vi "rs3 run_onchip_tare.vi"(0 "Device in":u64=2008212946240, 1 "Linux/Windows":u16(ring) items=["Linux (poling)", "Windows (interrupt)"], 2 "Auto Depth Preset\n(5 sec slower)":bool, 3 "On-Chip Calibration Mode":u16(ring) items=["Intrinsic", "Extrinsic"], 5 "ground truth, mm":sgl=500.0, 7 "Max step count (5-30)":u16=20, 9 "accuracy":u16(ring) items=["Very High (0.025%)", "High (0.05%)", "Medium (0.1%)", "Low (0.2%)"], 11 "error in (no error)":errorcluster, 12 "average step count (1-30)":u16=10, 13 "timeout ms":i32=8000) -> (4 "Device out":u64=2008212946240, 10 "error":u64, 14 "PointerToNewCalibrationTable":u64=2009804399744, 15 "error out":errorcluster)   [LabVIEW 2017, in "libRealSense3.lvlib"]
doc: "STARTS the streaming of a specific sensor, based on the input QUEUE."
uses:
  libRealSense3.lvlib
  realsense2.dll
panel:
  out "json":string="{\"average step count\": 10,\"step count\": 10, \"accuracy\": 0, \"scan parameter\": 0, \"data sampling\": 0}"
  # "RS Run On-Chip Tare"
  # "(C) 2019 Intel Corp.,  AGJ"
  # "[?1/?16/?2020 8:52 AM]  Angerman, Avishag:  \nstd::stringstream ss;\n        ss << \"{\\n \\\"speed\\\":\" << speed <<\n               \",\\n \\\"average_step_count\\\":\" << average_step_count <<\n               \",\\n \\\"step_count\\\":\" << step_count <<\n               \",\\n \\\"accuracy\\\":\" << accuracy <<\"}\"; \nthis is what I create on viewer , maybe you should try with \\n"
  # "std::stringstream ss;\n        ss << \"{\\n \\\"speed\\\":\" << speed <<\n               \",\\n \\\"average_step_count\\\":\" << average_step_count <<\n               \",\\n \\\"step_count\\\":\" << step_count <<\n               \",\\n \\\"accuracy\\\":\" << accuracy <<\"}\";"
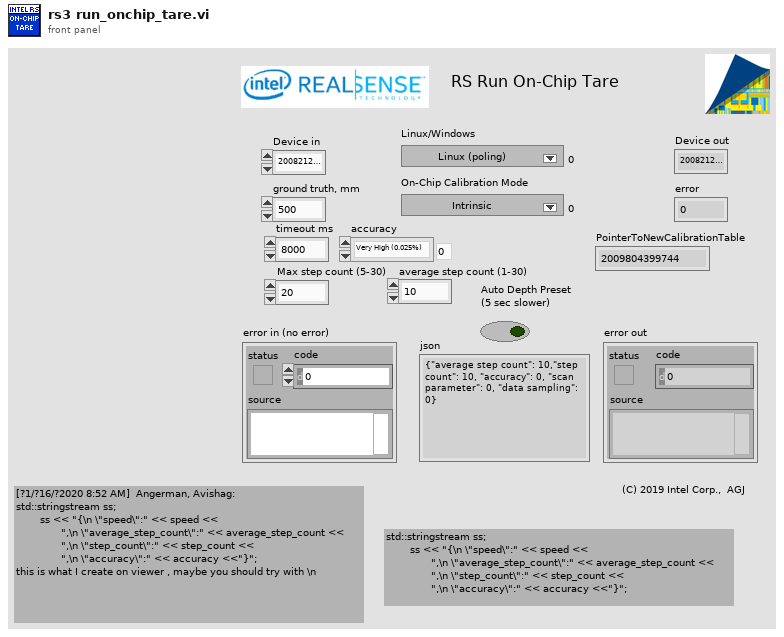
[diagram p1: front panel]
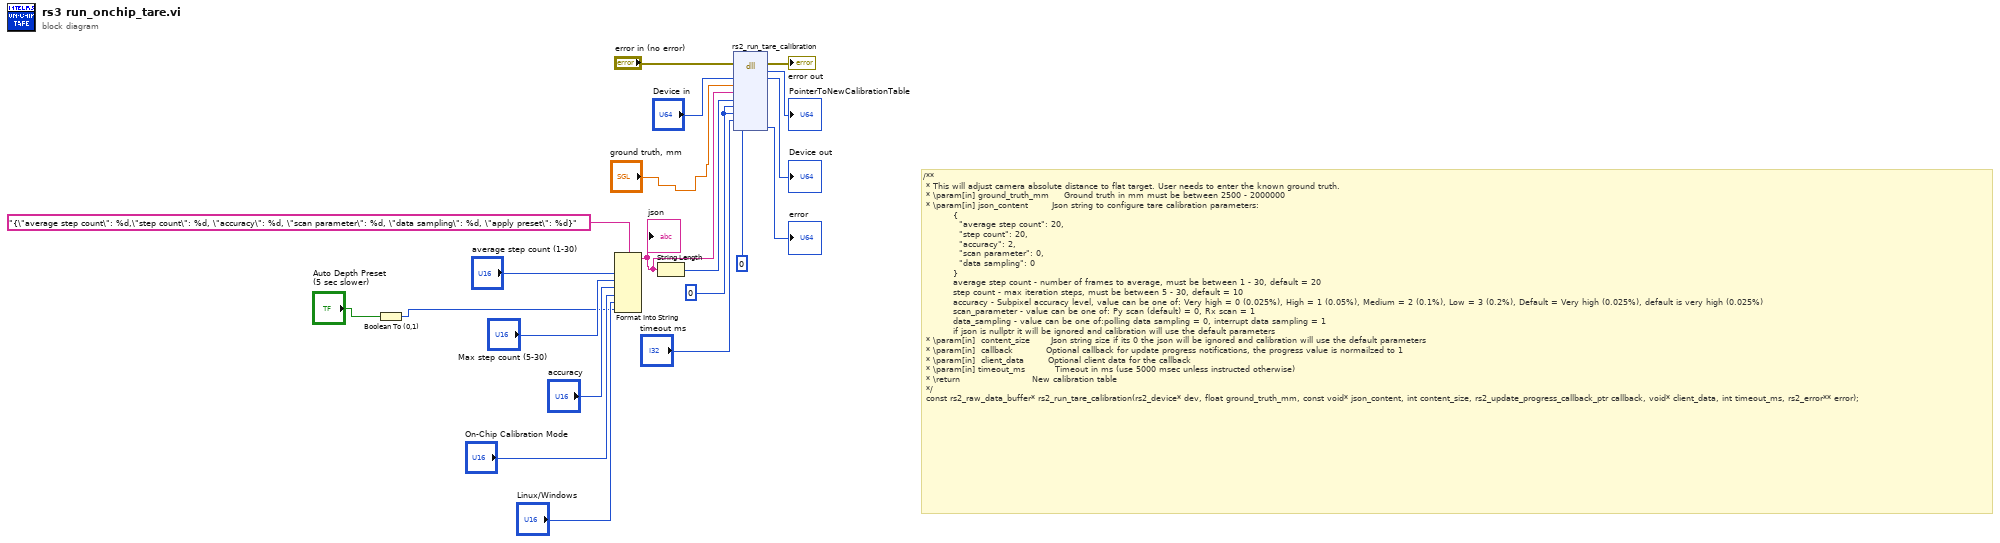
[diagram p0: block diagram]
diagram:
  w10 = u64 0 ("callback progress")
  # "/**\n\t* This will adjust camera absolute distance to flat target. User needs to enter the known ground truth.\n\t* \\param[in] ground_truth_mm     Ground truth in mm must be between 2500 - 2000000\n\t* \\param[in] json_content        Json string to configure tare calibration parameters:\n\t\t\t\t\t\t\t\t\t\t{\n\t\t\t\t\t\t\t\t\t\t  \"average step count\": 20,\n\t\t\t\t\t\t\t\t\t\t  \"step count\": 20,\n\t\t\t\t\t\t\t\t\t\t  \"accuracy\": 2,\n\t\t\t\t\t\t\t\t\t\t  \"scan parameter\": 0,\n\t\t\t\t\t\t\t\t\t\t  \"data sampling\": 0\n\t\t\t\t\t\t\t\t\t\t}\n\t\t\t\t\t\t\t\t\t\taverage step count - number of frames to average, must be between 1 - 30, default = 20\n\t\t\t\t\t\t\t\t\t\tstep count - max iteration steps, must be between 5 - 30, default = 10\n\t\t\t\t\t\t\t\t\t\taccuracy - Subpixel accuracy level, value can be one of: Very high = 0 (0.025%), High = 1 (0.05%), Medium = 2 (0.1%), Low = 3 (0.2%), Default = Very high (0.025%), default is very high (0.025%)\n\t\t\t\t\t\t\t\t\t\tscan_parameter - value can be one of: Py scan (default) = 0, Rx scan = 1\n\t\t\t\t\t\t\t\t\t\tdata_sampling - value can be one of:polling data sampling = 0, interrupt data sampling = 1\n\t\t\t\t\t\t\t\t\t\tif json is nullptr it will be ignored and calibration will use the default parameters\n\t* \\param[in]  content_size       Json string size if its 0 the json will be ignored and calibration will use the default parameters\n\t* \\param[in]  callback           Optional callback for update progress notifications, the progress value is normailzed to 1\n\t* \\param[in]  client_data        Optional client data for the callback\n\t* \\param[in] timeout_ms          Timeout in ms (use 5000 msec unless instructed otherwise)\n\t* \\return                        New calibration table\n\t*/\n\tconst rs2_raw_data_buffer* rs2_run_tare_calibration(rs2_device* dev, float ground_truth_mm, const void* json_content, int content_size, rs2_update_progress_callback_ptr callback, void* client_data, int timeout_ms, rs2_error** error);"
  n1 = Boolean To (0,1)(Boolean="Auto Depth Preset\n(5 sec slower)") -> (0, 1=w1:i16)
  n2 = Format Into String(format string="{\"average step count\": %d,\"step count\": %d, \"accuracy\": %d, \"scan parameter\": %d, \"data sampling\": %d, \"apply preset\": %d}", "average step count (1-30)", "Max step count (5-30)", "accuracy", "On-Chip Calibration Mode", "Linux/Windows", w1) -> (resulting string=w3:string)  [unwired: 2 in, 1 out]
  "json" <- w3
  n3 = String Length(string=w3) -> (length=w11:i32)
  n4 = dll-call lib="C:/Users/agrunnet/Documents/libRealSense6/realsense2.dll" fn="rs2_run_tare_calibration"(error in="error in (no error)", "device"="Device in", "Ground truth mm"="ground truth, mm", "json"=w3, "json content size"=w11, "callback progress"=w10, "client data"=w10, "timeout ms"="timeout ms", "error"=u64 0) -> (error out=→"error out":errorcluster, "calibrationTable"=→"PointerToNewCalibrationTable":u64, "device"=→"Device out":u64, "error"=→"error":u64)  [unwired: 8 in, 1 out]
